vi "Pump Calibration (sub vi).vi"(8 "error in (no error)":errorcluster, 9 "No. Solvents":u32, 10 "VISA Valve":refnum<visa-resource-name>, 11 "VISA Pump":refnum<visa-resource-name>) -> (0 "error out":errorcluster, 1 "Calibrated":bool, 2 "Polynomial Coefficients":dbl[][](array[numeric]))   [LabVIEW 2020]
uses:
  controls/Calibration State.ctl
  <vilib>/Analysis/6fits.llb/Curve Fitting Criteria.ctl
  <vilib>/Utility/file.llb/Read Delimited Spreadsheet (DBL).vi
  <vilib>/Utility/file.llb/Write Delimited Spreadsheet (DBL).vi
  <vilib>/Analysis/NI_AALPro.lvlib
panel:
  in  "Save Button":bool
  in  "Calculate":bool
  out "Display":string
  in  "Load":bool
  in  "Start":bool
  in  "Exit":bool
  in  "Measured Rates":dbl[][](array[numeric])
  in  "Test Rates":dbl[](array[numeric])
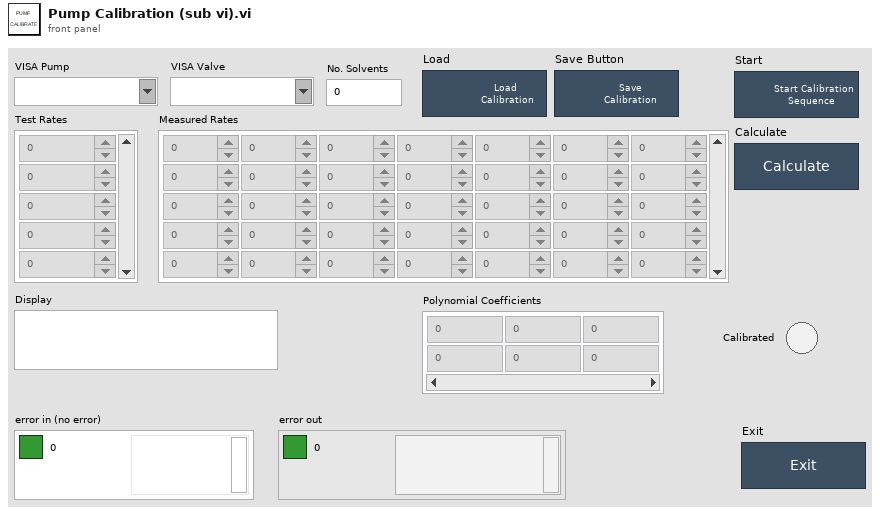
[diagram p1: front panel]
types:
  T1 = typedef "Calibration State.ctl" = enum16{"Initialise", "Wait for Event", "Calibration", "Calculate", "Save", "Load", "Exit"}
  T2 = typedef "NI_AALPro.lvlib/Curve Fitting Criteria.ctl" = u16
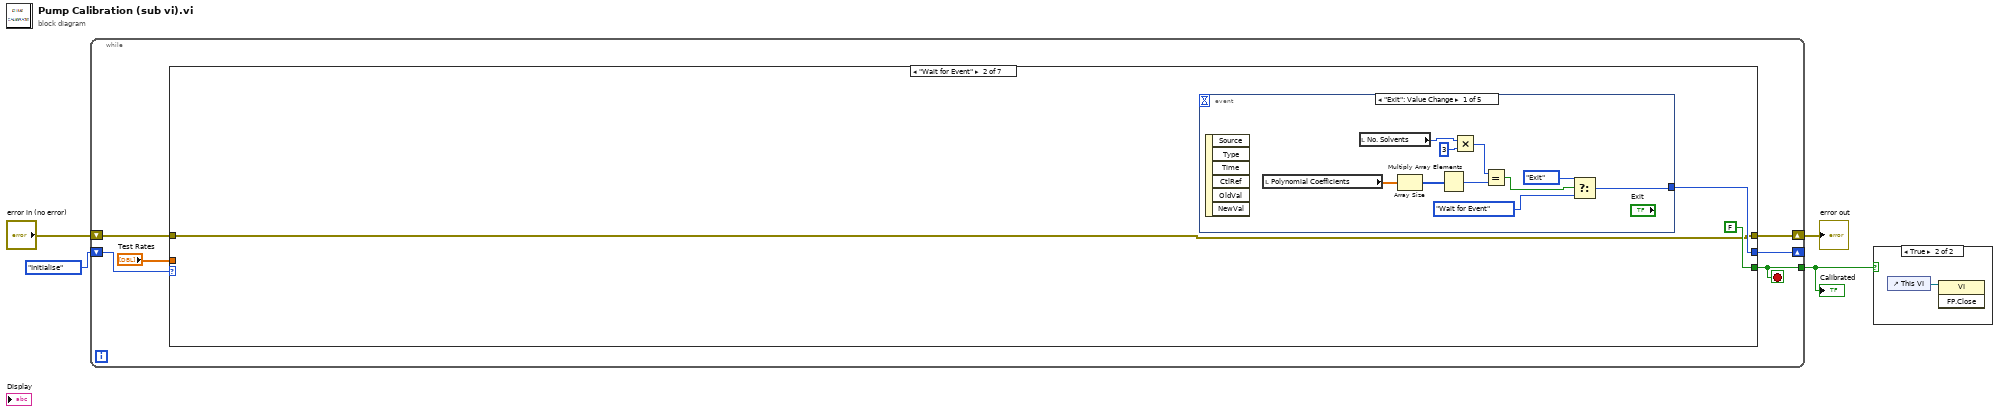
[diagram p0: block diagram]
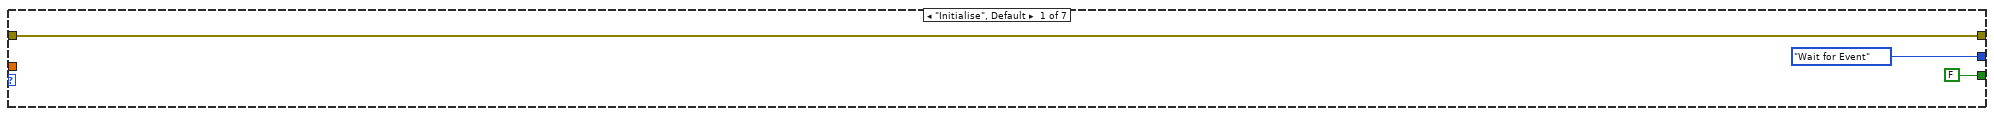
[diagram p3: hidden frame]
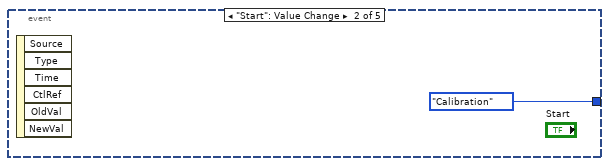
[diagram p4: hidden frame]
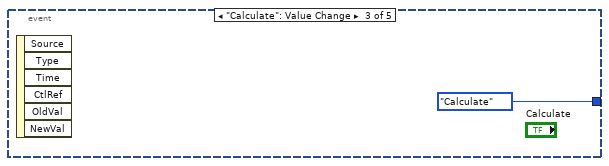
[diagram p5: hidden frame]
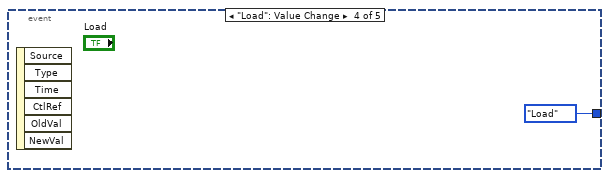
[diagram p6: hidden frame]
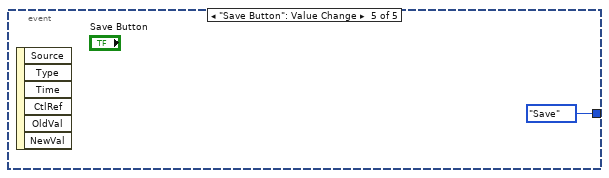
[diagram p7: hidden frame]
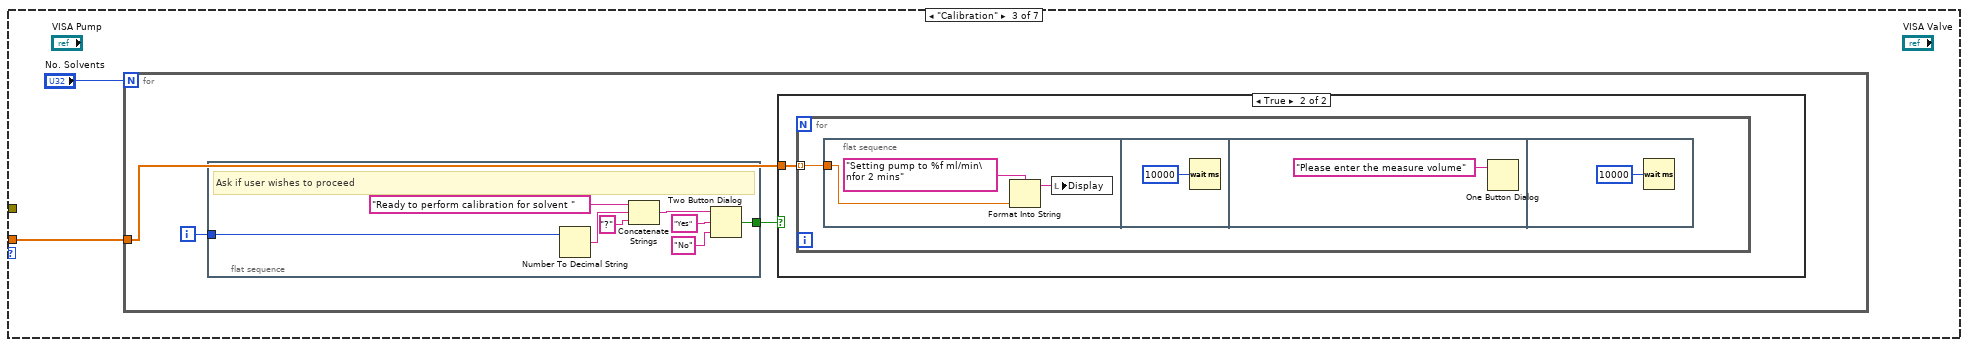
[diagram p8: hidden frame]
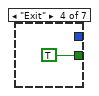
[diagram p10: hidden frame]
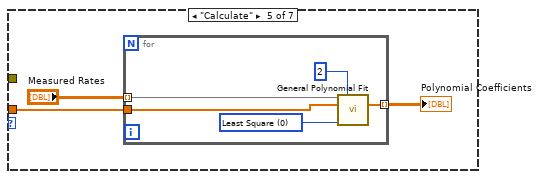
[diagram p11: hidden frame]
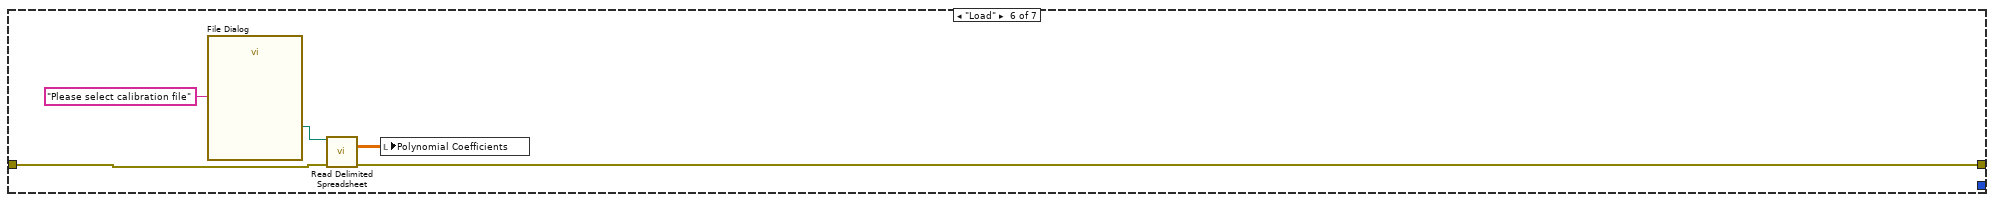
[diagram p12: hidden frame]
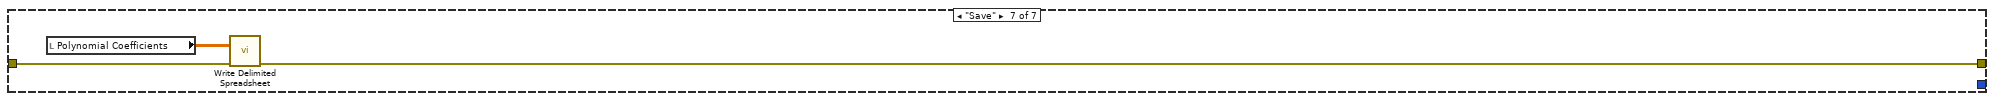
[diagram p13: hidden frame]
diagram:
  n1 = while {
    shift-right: [w9] -> _
    shift-left: Calibration_State."Initialise" -> [w10]
    shift-right: [w7] -> w2
    shift-left: "error in (no error)" -> [w8]
    tunnel: [w6] -> w1
    stop <- w6 stop-if-true
    n2 = case shown="\"Wait for Event\"" w10 {
      tunnel: "Test Rates" -> [_ _ w31 _ w54 _ _]
      tunnel: [Calibration_State."Wait for Event" w16 _ _ _ _ _] -> w9
      tunnel: [FALSE FALSE _ TRUE _ _ _] -> w6
      tunnel: w8 -> [w11 w14 _ _ _ w62 w67]
      tunnel: [w11 w14 _ _ _ w61 w66] -> w7
      frame "Initialise", Default {
      }
      frame "Wait for Event" {
        n3 = event shown="[0] \"Exit\": Value Change" {
          selector: _ -> [_ _ _ _ _]
          dyn-events: _ -> [_ _ _ _ _]
          timeout: _ -> [_ _ _ _ _]
          tunnel: [w17 Calibration_State."Calibration" Calibration_State."Calculate" Calibration_State."Load" Calibration_State."Save"] -> w16
          event "Exit": Value Change {
            n4 = event-data() -> ()  [unwired: 1 in, 6 out]
            n5 = local read "Polynomial Coefficients"() -> (w22:dbl[][])
            n6 = local read "No. Solvents"() -> (w26:u32)
            n7 = Array Size(array=w22) -> (size(s)=w21:i32[])
            n8 = Multiply Array Elements(1:w21) -> (0:w20:i32)
            n9 = Multiply(x=w26, y=u32 3) -> (x*y=w24:u32)
            n10 = Equal?(x=w24, y=w20) -> (x = y?=w23:bool)
            n11 = Select(t=Calibration_State."Exit", s=w23, f=Calibration_State."Wait for Event") -> (s? t:f=w17:T1)
          }
          event "Start": Value Change {
            n12 = event-data() -> ()  [unwired: 1 in, 6 out]
          }
          event "Calculate": Value Change {
            n13 = event-data() -> ()  [unwired: 1 in, 6 out]
          }
          event "Load": Value Change {
            n14 = event-data() -> ()  [unwired: 1 in, 6 out]
          }
          event "Save Button": Value Change {
            n15 = event-data() -> ()  [unwired: 1 in, 6 out]
          }
        }
      }
      frame "Calibration" {
        n16 = for {
          N: "No. Solvents" -> [_]
          tunnel: w31 -> [w34]
          i -> [w33]
          n17 = flat-sequence {
            tunnel: [w49] -> w35
            tunnel: w33 -> [w45]
            frame #0 {
              # "Ask if user wishes to proceed"
              n18 = Number To Decimal String(number=w45) -> (decimal integer string=w47:string)  [unwired: 1 in]
              n19 = Concatenate Strings("Ready to perform calibration for solvent " ("message"), w47, "?" ("string")) -> (w44:string)
              n20 = Two Button Dialog(message=w44, 1:"No" ("F button name (\"Cancel\")"), 2:"Yes" ("T button name (\"OK\")")) -> (T button?=w49:bool)
            }
          }
          n21 = case shown="True" w35 {
            tunnel: w34 -> [_ w36]
            frame False {
            }
            frame True {
              n22 = for {
                tunnel: w36 -> [w37] mode=indexing
                n23 = flat-sequence {
                  tunnel: w37 -> [w39]
                  frame #0 {
                    n24 = Format Into String(format string="Setting pump to %f ml/min\nfor 2 mins", w39) -> (resulting string=w38:string)  [unwired: 2 in, 1 out]
                    n25 = local write "Display"(w38) -> ()
                  }
                  frame #1 {
                    n26 = Wait (ms)(milliseconds to wait=u32 10000) -> ()  [unwired: 1 out]
                  }
                  frame #2 {
                    n27 = One Button Dialog(message="Please enter the measure volume") -> ()  [unwired: 1 in, 1 out]
                  }
                  frame #3 {
                    n28 = Wait (ms)(milliseconds to wait=u32 10000) -> ()  [unwired: 1 out]
                  }
                }
              }
            }
          }
        }
      }
      frame "Exit" {
      }
      frame "Calculate" {
        n29 = for {
          tunnel: w54 -> [w59]
          tunnel: "Measured Rates" -> [w57] mode=indexing
          tunnel: [w56] -> w53 mode=indexing
          w58 = T2 0 items=["Least Square", "Least Absolute Residual", "Bisquare"] ("method")
          n30 = call <vilib>:"General Polynomial Fit.vi"("Y"=w57, "polynomial order"=2, "X"=w59, "method"=w58) -> ("Polynomial Coefficients"=w56:dbl[])  [unwired: 8 in, 3 out]
        }
        "Polynomial Coefficients" <- w53
      }
      frame "Load" {
        n31 = call "File Dialog"("prompt"="Please select calibration file") -> ("selected path"=w64:path)  [unwired: 11 in, 3 out]
        n32 = call-poly <vilib>:"Read Delimited Spreadsheet.vi"("file path (dialog if empty)"=w64, "error in (no error)"=w62) -> ("all rows"=w63:dbl[][], "error out"=w61:errorcluster)  [unwired: 8 in, 4 out]
        n33 = local write "Polynomial Coefficients"(w63) -> ()
      }
      frame "Save" {
        n34 = local read "Polynomial Coefficients"() -> (w68:dbl[][])
        n35 = call-poly <vilib>:"Write Delimited Spreadsheet.vi"("2D data"=w68, "error in (no error)"=w67) -> ("error out"=w66:errorcluster)  [unwired: 12 in, 1 out]
      }
    }
  }
  "error out" <- w2
  "Calibrated" <- w1
  n36 = case shown="True" w1 {
    frame False {
    }
    frame True {
      n37 = control-ref of="This VI"() -> (w69:refnum<vi>)
      n38 = invoke class="VI" method="FP.Close"(reference=w69) -> ()  [unwired: 2 in, 3 out]
    }
  }
